vi "LorentzianRCfilter.vi"(3 "output control":T1, 4 "data":T2, 5 "X":dbl[](array[numeric]), 6 "a":dbl[](array[numeric])) -> (0 "error out":errorcluster, 1 "f'(X,a)":dbl[][](array[numeric]), 2 "f(X,a)":dbl[](array[numeric]))   [LabVIEW 2010]
doc: "This template is the starting point for creating a model function to be passed to the Nonlinear Curve Fit.vi."
uses:
  <vilib>/gmath/NumericalOptimization/objective function data.ctl
  <vilib>/gmath/NumericalOptimization/LM_output select.ctl
  <vilib>/gmath/NI_Gmath.lvlib
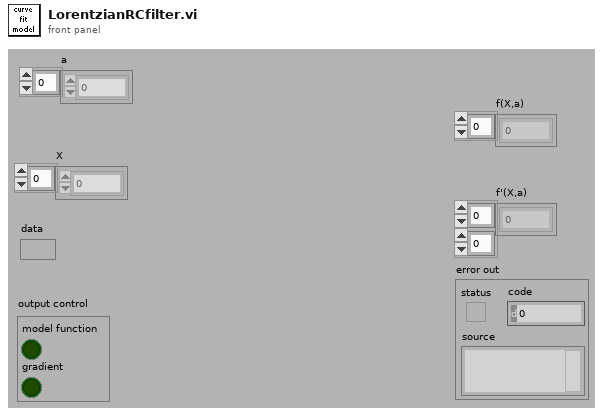
[diagram p1: front panel]
types:
  T1 = typedef "NI_Gmath.lvlib/LM_output select.ctl" = cluster{"model function":bool, "gradient":bool}
  T2 = typedef "NI_Gmath.lvlib/objective function data.ctl" = variant
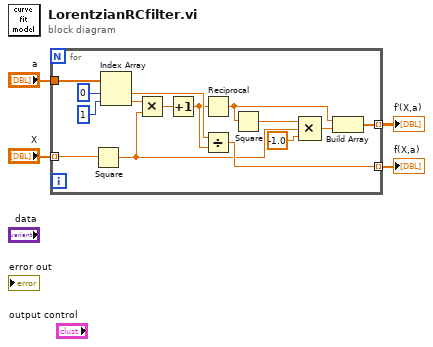
[diagram p0: block diagram]
diagram:
  n1 = for {
    tunnel: "a" -> [w19]
    tunnel: "X" -> [w15] mode=indexing
    tunnel: [w18] -> w2 mode=indexing
    tunnel: [w11] -> w1 mode=indexing
    n2 = Square(x=w15) -> (x^2=w7:dbl)
    n3 = Index Array(array=w19, index #1=0 ("index"), index #2=1 ("index")) -> (element #1=w12:dbl, element #2=w14:dbl)
    n4 = Multiply(x=w14, y=w7) -> (x*y=w13:dbl)
    n5 = Increment(x=w13) -> (x+1=w10:dbl)
    n6 = Reciprocal(x=w10) -> (1/x=w9:dbl)
    n7 = Divide(x=w12, y=w10) -> (x/y=w11:dbl)
    n8 = Square(x=w9) -> (x^2=w6:dbl)
    n9 = Compound Arithmetic op=MULTIPLY(w6, w7, -1.0 ("value")) -> (w8:dbl)
    n10 = Build Array(w9, w8) -> (w18:dbl[])
  }
  "f(X,a)" <- w1
  "f'(X,a)" <- w2
